vi "扫描绘制.vi"(7 "完成":bool, 8 "曲线设置":T1, 10 "历史数据":cluster{"数据":dbl[][]}[](array[cluster]), 11 "映射方式":T2) -> (0 "曲线属性":cluster{"曲线名":string, "曲线颜色":u32, "线条宽度":u8}[](array[cluster]), 3 "XY图":cluster{"数据":dbl[], "数据":dbl[]}[](array[cluster]))   [LabVIEW 2020, in "数据显示.xctl"]
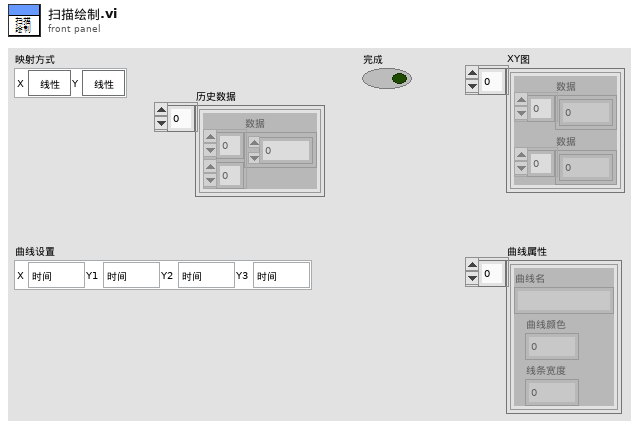
[diagram p1: front panel]
types:
  T1 = typedef "数据显示.xctl/曲线设置.ctl" = cluster{"X":enum16{"时间", "设置电压", "读取电流", "读取电压"}, "Y1":enum16{"时间", "设置电压", "读取电流", "读取电压"}, "Y2":enum16{"时间", "设置电压", "读取电流", "读取电压", "无"}, "Y3":enum16{"时间", "设置电压", "读取电流", "读取电压", "无"}}
  T2 = typedef "数据显示.xctl/映射方式.ctl" = cluster{"X":bool, "Y":bool}
  T3 = cluster{"output string":string, "曲线颜色":u32, "线条宽度":u8}
  T4 = cluster{"output string":string, "曲线颜色":u32, "线条宽度":u8}[]
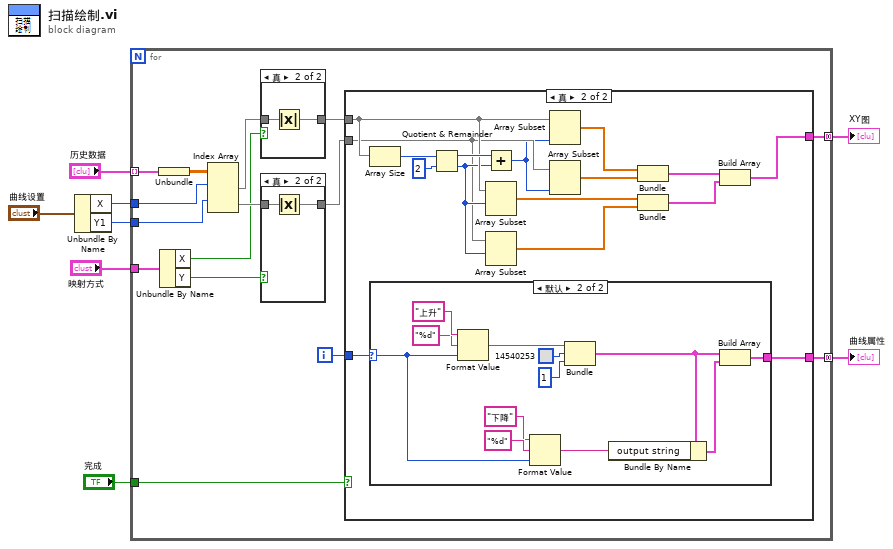
[diagram p0: block diagram]
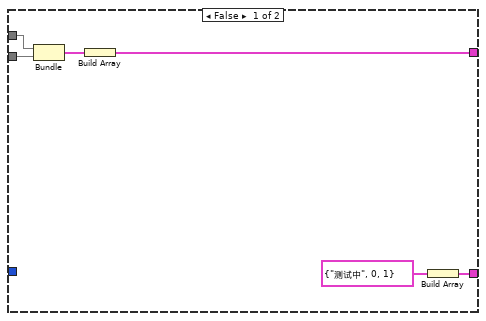
[diagram p2: hidden frame]
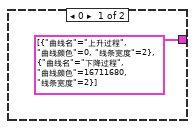
[diagram p3: hidden frame]
diagram:
  n1 = Unbundle By Name("曲线设置") -> ("X"=w4:enum16{"时间", "设置电压", "读取电流", "读取电压"}, "Y1"=w5:enum16{"时间", "设置电压", "读取电流", "读取电压"})
  n2 = for {
    tunnel: w5 -> [w23]
    tunnel: w4 -> [w22]
    tunnel: [w19] -> w8 mode=concatenating
    tunnel: "映射方式" -> [w18]
    tunnel: "历史数据" -> [w17] mode=indexing
    tunnel: "完成" -> [w9]
    tunnel: [w11] -> w1 mode=concatenating
    i -> [w10]
    n3 = Unbundle(w17) -> ("数据"=w16:dbl[][])
    n4 = Unbundle By Name(w18) -> ("X"=w15:bool, "Y"=w12:bool)
    n5 = Index Array(array=w16, index (row) #1=w22, index (row) #2=w23) -> (element #1=w20:dbl[], element #2=w21:dbl[])  [unwired: 2 in]
    n6 = case shown="真" w15 {
      tunnel: w20 -> [w59 w61]
      tunnel: [w59 w60] -> w14
      frame False {
      }
      frame True {
        n7 = Absolute Value(x=w61) -> (abs(x)=w60:dbl[])
      }
    }
    n8 = case shown="真" w12 {
      tunnel: w21 -> [w62 w64]
      tunnel: [w62 w63] -> w13
      frame False {
      }
      frame True {
        n9 = Absolute Value(x=w64) -> (abs(x)=w63:dbl[])
      }
    }
    n10 = case shown="真" w9 {
      tunnel: [w26 w45] -> w19
      tunnel: w14 -> [w28 w39]
      tunnel: w13 -> [w27 w34]
      tunnel: [w24 w30] -> w11
      tunnel: w10 -> [_ w31]
      frame False {
        n11 = Bundle("数据"=w28, "数据"=w27) -> (w29:cluster{"数据":dbl[], "数据":dbl[]})  [unwired: 1 in]
        n12 = Build Array(w29) -> (w26:cluster{"数据":dbl[], "数据":dbl[]}[])
        n13 = Build Array(cluster{"曲线名":string, "曲线颜色":u32, "线条宽度":u8} {"曲线名"="测试中", "曲线颜色"=0, "线条宽度"=1} ("曲线属性")) -> (w24:cluster{"曲线名":string, "曲线颜色":u32, "线条宽度":u8}[])
      }
      frame True {
        n14 = Array Size(array=w39) -> (size(s)=w41:i32)
        n15 = case shown="默认" w31 {
          selector: w31 -> [_ w51]
          tunnel: [cluster{"曲线名":string, "曲线颜色":u32, "线条宽度":u8}[] [{"曲线名"="上升过程", "曲线颜色"=0, "线条宽度"=2}, {"曲线名"="下降过程", "曲线颜色"=16711680, "线条宽度"=2}] ("添加的数组") w47] -> w30
          frame 0 {
          }
          frame Default {
            n16 = Format Value(string ("")="上升" ("曲线名"), format string="%d" ("格式字符串"), value (0)=w51) -> (output string=w54:string)
            n17 = Format Value(string ("")="下降" ("曲线名"), format string="%d" ("格式字符串"), value (0)=w51) -> (output string=w50:string)
            n18 = Bundle("output string"=w54, "曲线颜色"=u32 14540253, "线条宽度"=u8 1) -> (w49:T3)  [unwired: 1 in]
            n19 = Bundle By Name(cluster=w49, "output string"=w50) -> (w48:T3)
            n20 = Build Array(w49, w48) -> (w47:T4)
          }
        }
        n21 = Quotient & Remainder(x=w41, y=2) -> (x-y*floor(x/y)=w40:i32, floor(x/y)=w36:i32)
        n22 = Add(x=w40, y=w36) -> (x+y=w33:i32)
        n23 = Array Subset(array=w39, index=w36) -> (w37:dbl[])  [unwired: 1 in]
        n24 = Array Subset(array=w34, index=w36) -> (w35:dbl[])  [unwired: 1 in]
        n25 = Array Subset(array=w39, length=w33) -> (w38:dbl[])  [unwired: 1 in]
        n26 = Array Subset(array=w34, length=w33) -> (w32:dbl[])  [unwired: 1 in]
        n27 = Bundle(w38, w32) -> (w44:cluster{dbl[], dbl[]})  [unwired: 1 in]
        n28 = Bundle(w37, w35) -> (w43:cluster{dbl[], dbl[]})  [unwired: 1 in]
        n29 = Build Array(w44, w43) -> (w45:cluster{dbl[], dbl[]}[])
      }
    }
  }
  "曲线属性" <- w1
  "XY图" <- w8
